vi "add_timetraces_overlay.vi"(8 "error in (no error)":errorcluster, 9 "filenames":string[](array[string]), 10 "map size":cluster{dbl, dbl, dbl, dbl}, 11 "Refnum in":T2) -> (0 "error out":errorcluster, 2 "Timetraces":T1(array[cluster]), 3 "Refnum out":T2)   [LabVIEW 2012]
uses:
  <vilib>/vision/Image Controls.llb/IMAQ Image.ctl
  <vilib>/regexp/Match Regular Expression.xnode
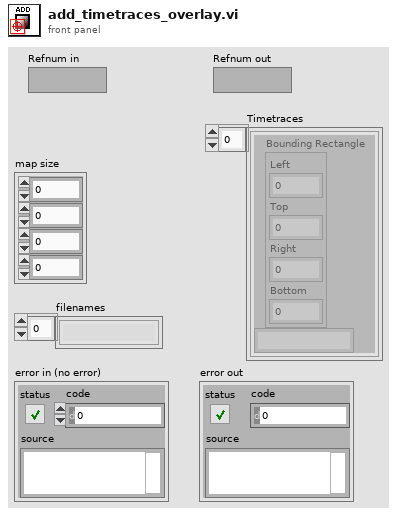
[diagram p1: front panel]
types:
  T1 = cluster{"Bounding Rectangle":cluster{"Left":i32, "Top":i32, "Right":i32, "Bottom":i32}, string}[]
  T2 = typedef "IMAQ Image.ctl" = refnum<image>
  T3 = cluster{"Left":i32, "Top":i32, "Right":i32, "Bottom":i32}
  T4 = cluster{"Bounding Rectangle":cluster{"Left":i32, "Top":i32, "Right":i32, "Bottom":i32}, string}
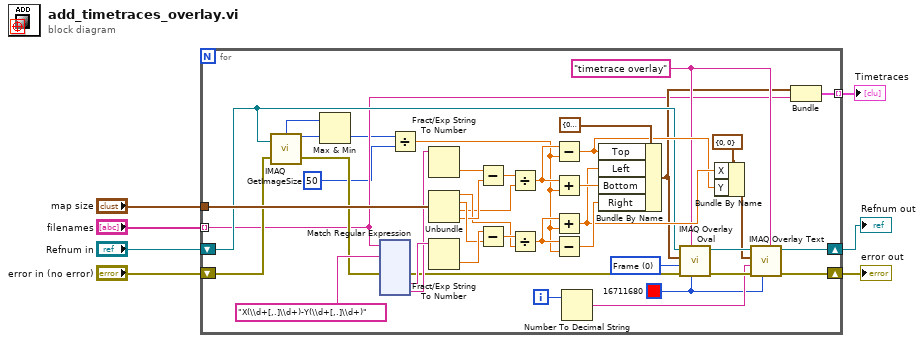
[diagram p0: block diagram]
diagram:
  n1 = for {
    tunnel: "filenames" -> [w14] mode=indexing
    tunnel: "map size" -> [w49]
    shift-right: [w28] -> w6
    shift-left: "Refnum in" -> [w18]
    shift-right: [w27] -> w7
    shift-left: "error in (no error)" -> [w17]
    tunnel: [w13] -> w1 mode=indexing
    i -> [w22]
    w19 = "timetrace overlay" ("Group")
    w20 = u32 16711680 ("Color")
    w36 = u32 0 items=["Frame", "Fill"] ("Drawing Mode (Frame)")
    n2 = call "IMAQ GetImageSize"("Image"=w18, "error in (no error)"=w17) -> ("Y Resolution"=w11:i32, "X Resolution"=w12:i32, "error out"=w16:errorcluster)  [unwired: 2 in]
    n3 = Max & Min(x=w12, y=w11) -> (min(x,y)=w10:i32)  [unwired: 1 out]
    n4 = xnode "Match Regular Expression"("input string"=w14, "regular expression"="X(\\d+[,.]\\d+)-Y(\\d+[,.]\\d+)", "error in"=w16) -> ("error out"=w37:errorcluster, "submatch 1"=w47:string, "submatch 2"=w46:string)  [unwired: 3 in, 4 out]
    n5 = Divide(x=w10, y=50) -> (x/y=w8:dbl)
    n6 = Fract/Exp String To Number(string=w46) -> (number=w43:dbl)  [unwired: 3 in, 1 out]
    n7 = Unbundle(w49) -> (w39:dbl, w44:dbl, w38:dbl, w42:dbl)
    n8 = Fract/Exp String To Number(string=w47) -> (number=w45:dbl)  [unwired: 3 in, 1 out]
    n9 = Subtract(x=w43, y=w42) -> (x-y=w40:dbl)
    n10 = Subtract(x=w45, y=w44) -> (x-y=w41:dbl)
    n11 = Divide(x=w40, y=w38) -> (x/y=w33:dbl)
    n12 = Divide(x=w41, y=w39) -> (x/y=w31:dbl)
    n13 = Subtract(x=w33, y=w8) -> (x-y=w23:dbl)
    n14 = Add(x=w33, y=w8) -> (x+y=w32:dbl)
    n15 = Add(x=w31, y=w8) -> (x+y=w24:dbl)
    n16 = Subtract(x=w31, y=w8) -> (x-y=w34:dbl)
    n17 = Number To Decimal String(number=w22) -> (decimal integer string=w21:string)  [unwired: 1 in]
    n18 = Bundle By Name(cluster=T3 {"Left"=0, "Top"=0, "Right"=0, "Bottom"=0} ("Bounding Rectangle"), "Top"=w23, "Left"=w24, "Bottom"=w32, "Right"=w34) -> (w15:T3)
    n19 = call "IMAQ Overlay Oval"("Color"=w20, "Group"=w19, "error in (no error)"=w37, "Drawing Mode (Frame)"=w36, "Bounding Rectangle"=w15, "Image"=w18) -> ("error out"=w29:errorcluster, "Image Out"=w30:T2)  [unwired: 4 in]
    n20 = Bundle By Name(cluster=cluster{"X":i32, "Y":i32} {"X"=0, "Y"=0} ("Origin"), "X"=w24, "Y"=w23) -> (w25:cluster{"X":i32, "Y":i32})
    n21 = call "IMAQ Overlay Text"("Group"=w19, "Text Color (black)"=w20, "error in (no error)"=w29, "String"=w21, "Origin"=w25, "Image"=w30) -> ("error out"=w27:errorcluster, "Image Out"=w28:T2)  [unwired: 4 in]
    n22 = Bundle("Bounding Rectangle"=w15, w14) -> (w13:T4)  [unwired: 1 in]
  }
  "error out" <- w7
  "Refnum out" <- w6
  "Timetraces" <- w1
